vi "Grados.vi"(5 "error in (no error)":errorcluster, 6 "Unidad":enum16{"C", "K", "F"}(ring), 7 "Grados":dbl) -> (0 "error out":errorcluster, 1 "Farenheit":dbl, 2 "Kelvin":dbl, 3 "Centigrados":dbl)   [LabVIEW 2020]
panel:
  in  "RETURN":bool
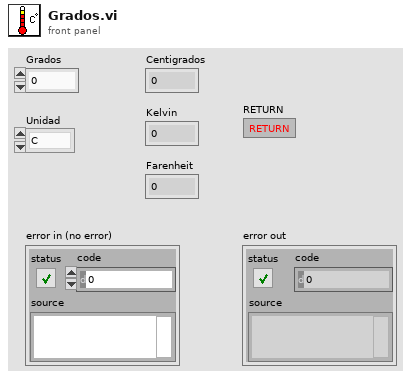
[diagram p1: front panel]
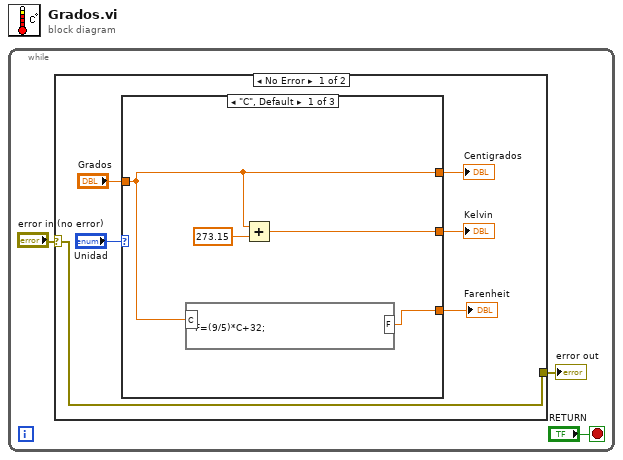
[diagram p0: block diagram]
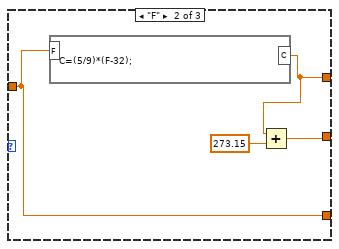
[diagram p2: hidden frame]
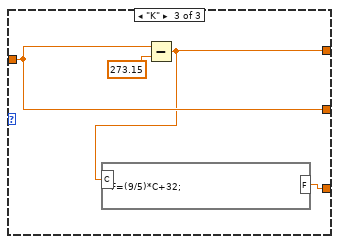
[diagram p3: hidden frame]
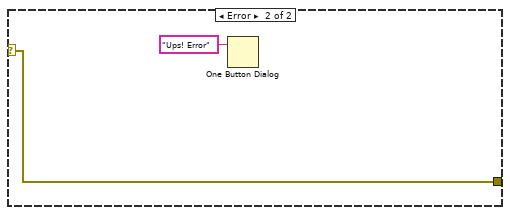
[diagram p4: hidden frame]
diagram:
  n1 = while {
    stop <- "RETURN" stop-if-true
    n2 = case shown="No Error" "error in (no error)" {
      selector: "error in (no error)" -> [w4 w22]
      tunnel: [w4 w22] -> w2
      frame No Error {
        n3 = case shown="\"C\", Default" "Unidad" {
          tunnel: "Grados" -> [w11 w17 w20]
          tunnel: [w11 w16 w19] -> w7
          tunnel: [w12 w15 w20] -> w6
          tunnel: [w13 w17 w18] -> w5
          frame "C", Default {
            n4 = formula code="F=(9/5)*C+32;"("C"=w11) -> ("F"=w13:dbl)
            n5 = Add(x=w11, y=273.15) -> (x+y=w12:dbl)
          }
          frame "F" {
            n6 = formula code="C=(5/9)*(F-32);"("F"=w17) -> ("C"=w16:dbl)
            n7 = Add(x=w16, y=273.15) -> (x+y=w15:dbl)
          }
          frame "K" {
            n8 = Subtract(x=w20, y=273.15) -> (x-y=w19:dbl)
            n9 = formula code="F=(9/5)*C+32;"("C"=w19) -> ("F"=w18:dbl)
          }
        }
        "Centigrados" <- w7
        "Kelvin" <- w6
        "Farenheit" <- w5
      }
      frame Error {
        n10 = One Button Dialog(message="Ups! Error") -> ()  [unwired: 1 in, 1 out]
      }
    }
    "error out" <- w2
  }
